vi "ContextHelp_StartUpTask.vi"(1 "CallerRef":refnum<vi>, 2 "HelpReference":refnum<vi>, 5 "error in (no error)":errorcluster) -> (14 "PopUpTaskEvent":T1, 19 "error out":errorcluster)   [LabVIEW 2010]
uses:
  ContextHelp_EventType.ctl
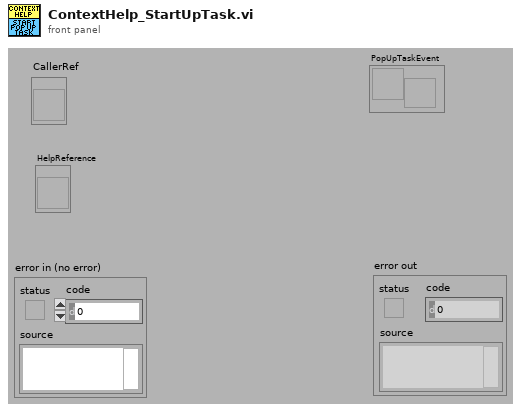
[diagram p1: front panel]
types:
  T1 = typedef "ContextHelp_EventType.ctl" = refnum<user-event>
  T2 = enum32{"Bad", "Idle", "Run top level", "Running"}
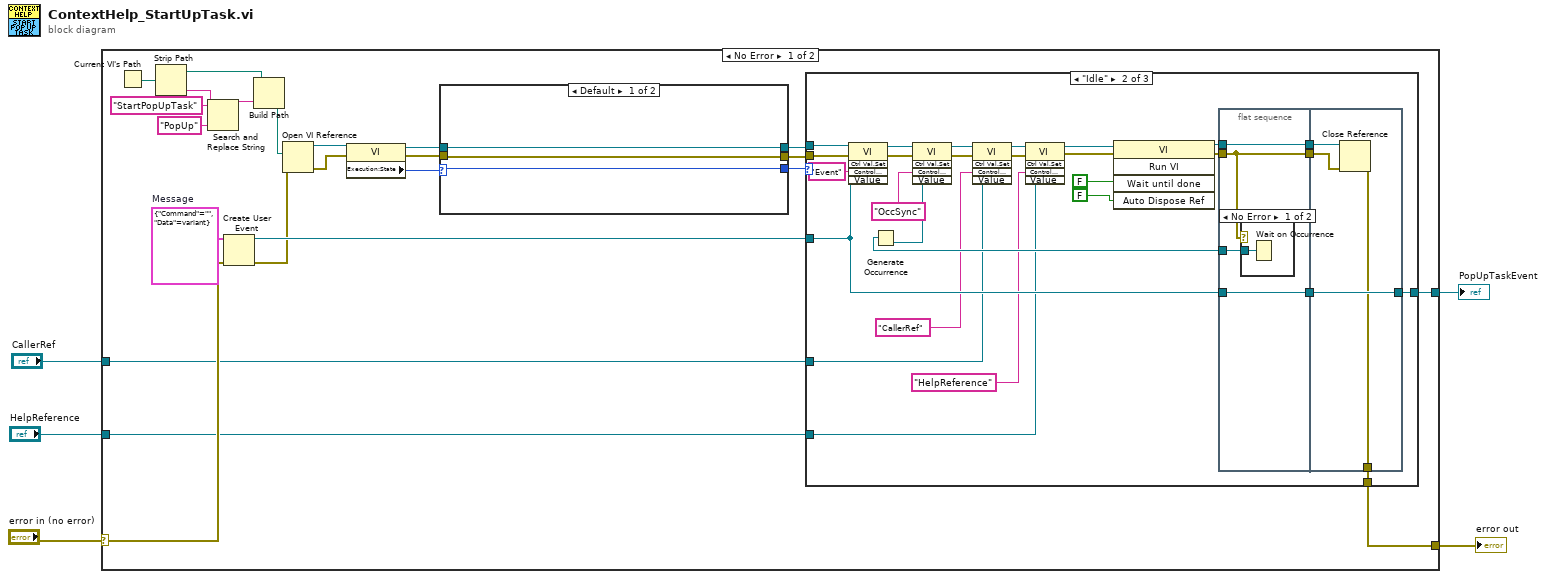
[diagram p0: block diagram]
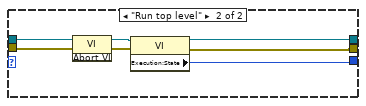
[diagram p2: hidden frame]
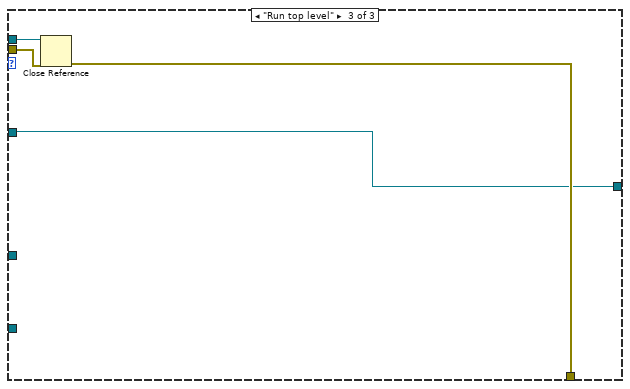
[diagram p5: hidden frame]
diagram:
  n1 = case shown="No Error" "error in (no error)" {
    selector: "error in (no error)" -> [w16 w81]
    tunnel: [w19 _] -> w5
    tunnel: [w18 w81] -> w4
    tunnel: "CallerRef" -> [w7 _]
    tunnel: "HelpReference" -> [w6 _]
    frame No Error {
      w21 = cluster{"Command":string, "Data":variant} {"Command"="", "Data"=variant}  # Message
      n2 = Current VI's Path() -> (path=w28:path)
      n3 = Strip Path(path=w28) -> (stripped path=w23:path, name=w27:string)
      n4 = Search and Replace String(input string=w27, search string="StartPopUpTask", replace string="PopUp" ("replace string (\"\")")) -> (result string=w24:string)  [unwired: 1 in, 7 out]
      n5 = Create User Event(user event datatype=w21, error in=w16) -> (user event=w20:refnum<user-event>, error out=w17:errorcluster)
      n6 = Build Path(base path=w23, name or relative path=w24) -> (appended path=w22:path)
      n7 = Open VI Reference(vi path=w22, error in (no error)=w17) -> (vi reference=w15:refnum<vi>, error out=w14:errorcluster)  [unwired: 4 out]
      n8 = property class="VI"(reference=w15, error in=w14) -> (reference out=w13:refnum<vi>, error out=w12:errorcluster, "Execution:State"=w11:T2)
      n9 = case shown="Default" w11 {
        selector: w11 -> [w31 _]
        tunnel: w13 -> [w29 w38]
        tunnel: w12 -> [w30 w37]
        tunnel: [w31 w34] -> w10
        tunnel: [w30 w32] -> w9
        tunnel: [w29 w33] -> w8
        frame Default {
        }
        frame "Run top level" {
          n10 = invoke class="VI" method="Abort VI"(reference=w38, error in=w37) -> (reference out=w36:refnum<vi>, error out=w35:errorcluster)  [unwired: 1 in, 1 out]
          n11 = property class="VI"(reference=w36, error in=w35) -> (reference out=w33:refnum<vi>, error out=w32:errorcluster, "Execution:State"=w34:T2)
        }
      }
      n12 = case shown="\"Idle\"" w10 {
        tunnel: w8 -> [_ w64 w80]
        tunnel: w9 -> [w39 w63 w79]
        tunnel: w20 -> [w40 w53 w77]
        tunnel: [w40 w52 w77] -> w19
        tunnel: [w39 w51 w78] -> w18
        tunnel: w7 -> [_ w47 _]
        tunnel: w6 -> [_ w41 _]
        frame "Bad", Default {
        }
        frame "Idle" {
          n13 = invoke class="VI" method="Ctrl Val.Set"(reference=w64, error in=w63, "Control Name"="Event", "Value"=w53) -> (reference out=w57:refnum<vi>, error out=w56:errorcluster)  [unwired: 1 in, 3 out]
          n14 = Generate Occurrence() -> (w54:refnum<k4>)
          n15 = invoke class="VI" method="Ctrl Val.Set"(reference=w57, error in=w56, "Control Name"="OccSync", "Value"=w54) -> (reference out=w50:refnum<vi>, error out=w49:errorcluster)  [unwired: 1 in, 3 out]
          n16 = invoke class="VI" method="Ctrl Val.Set"(reference=w50, error in=w49, "Control Name"="CallerRef", "Value"=w47) -> (reference out=w46:refnum<vi>, error out=w45:errorcluster)  [unwired: 1 in, 3 out]
          n17 = invoke class="VI" method="Ctrl Val.Set"(reference=w46, error in=w45, "Control Name"="HelpReference", "Value"=w41) -> (reference out=w44:refnum<vi>, error out=w43:errorcluster)  [unwired: 1 in, 3 out]
          n18 = invoke class="VI" method="Run VI"(reference=w44, error in=w43, "Wait until done"=FALSE, "Auto Dispose Ref"=FALSE) -> (reference out=w59:refnum<vi>, error out=w58:errorcluster)  [unwired: 1 in, 3 out]
          n19 = flat-sequence {
            tunnel: w53 -> [w70]
            tunnel: w58 -> [w68]
            tunnel: w59 -> [w71]
            tunnel: [w71] -> w67
            tunnel: [w68] -> w66
            tunnel: [w70] -> w65
            tunnel: w54 -> [w69]
            tunnel: w67 -> [w76]
            tunnel: w66 -> [w75]
            tunnel: w65 -> [w74]
            tunnel: [w74] -> w52
            tunnel: [w73] -> w51
            frame #0 {
              n20 = case shown="No Error" w68 {
                tunnel: w69 -> [w72 _]
                frame No Error {
                  n21 = Wait on Occurrence(2:w72) -> ()  [unwired: 3 out]
                }
                frame Error {
                }
              }
            }
            frame #1 {
              n22 = Close Reference(reference=w76, error in (no error)=w75) -> (error out=w73:errorcluster)
            }
          }
        }
        frame "Run top level" {
          n23 = Close Reference(reference=w80, error in (no error)=w79) -> (error out=w78:errorcluster)
        }
      }
    }
    frame Error {
    }
  }
  "PopUpTaskEvent" <- w5
  "error out" <- w4
